vi "TriggerConfg.vi"(0 "VISA IN":refnum<visa-resource-name>, 1 "Trigger Mode":string(combo)="CONTinuous", 2 "Groups Count":i32=1, 3 "All Points? ON/OFF":bool=TRUE, 5 "error in":errorcluster, 6 "Channel":i32=1) -> (14 "VISA Out":refnum<visa-resource-name>, 19 "error out":errorcluster)   [LabVIEW 2018, in "PNA-X.lvlib"]
uses:
  PNA-X.lvlib
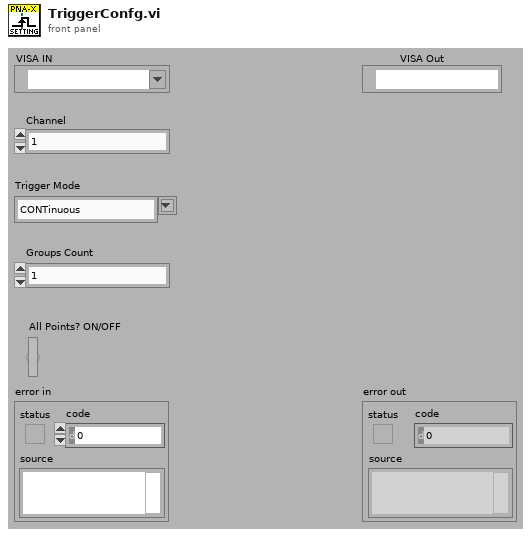
[diagram p1: front panel]
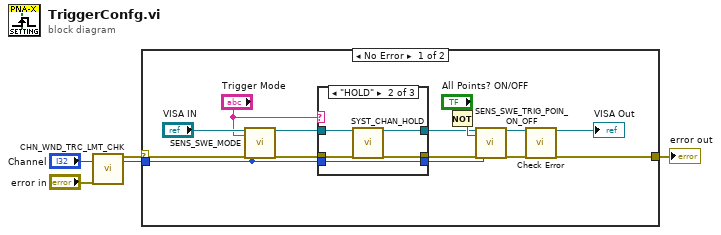
[diagram p0: block diagram]
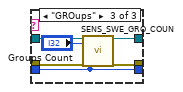
[diagram p3: hidden frame]
diagram:
  n1 = call "CHN_WND_TRC_LMT_CHK.vi"("Channel"="Channel", "error in"="error in") -> ("error out"=w2:errorcluster, "Channel"=w1:i32)  [unwired: 13 in, 3 out]
  n2 = case shown="No Error" w2 {
    selector: w2 -> [w8 w36]
    tunnel: [w19 w35] -> w4
    tunnel: w1 -> [w7 _]
    frame No Error {
      n3 = call "SENS_SWE_MODE.vi"("VISA IN"="VISA IN", "Trigger Mode"="Trigger Mode", "error in"=w8, "Channel"=w7) -> ("VISA Out"=w17:refnum<visa-resource-name>, "error out"=w15:errorcluster)  [unwired: 14 in]
      n4 = case shown="\"HOLD\"" "Trigger Mode" {
        tunnel: w17 -> [w23 w25 w32]
        tunnel: w15 -> [w22 w28 w34]
        tunnel: [w23 w26 w31] -> w10
        tunnel: [w22 w27 w33] -> w9
        tunnel: w7 -> [w21 w24 w29]
        tunnel: [w21 w24 w29] -> w6
        frame Default {
        }
        frame "HOLD" {
          n5 = call "SYST_CHAN_HOLD.vi"("VISA IN"=w25, "error in"=w28) -> ("VISA Out"=w26:refnum<visa-resource-name>, "error out"=w27:errorcluster)  [unwired: 16 in]
        }
        frame "GROups" {
          n6 = call "SENS_SWE_GRO_COUN.vi"("VISA IN"=w32, "Count"="Groups Count", "error in"=w34, "Channel"=w29) -> ("VISA Out"=w31:refnum<visa-resource-name>, "error out"=w33:errorcluster)  [unwired: 14 in]
        }
      }
      n7 = Not(x="All Points? ON/OFF") -> (.not. x?=w13:bool)
      n8 = call "SENS_SWE_TRIG_POIN_ON_OFF.vi"("VISA IN"=w10, "One data point? ON/OFF"=w13, "error in"=w9, "Channel"=w6) -> ("VISA Out"=w16:refnum<visa-resource-name>, "error out"=w14:errorcluster)  [unwired: 14 in]
      n9 = call "Check Error.vi"("VISA Resource Name"=w16, "error in (no error)"=w14) -> ("dup VISA session"=→"VISA Out":refnum<visa-resource-name>, "error out"=w19:errorcluster)  [unwired: 16 in]
    }
    frame Error {
      n10 = call <vilib>:"Simple Error Handler.vi"("error in (no error)"=w36) -> ("error out"=w35:errorcluster)  [unwired: 4 in, 4 out]
    }
  }
  "error out" <- w4
